vi "niRFUtil CONV Bit Stream to Number.vi"(3 "Length":i32 max=32, 4 "Index":i32, 5 "Bit Stream In":T1 min=0) -> (1 "Number":u32 max=16777215 format="%.0x", 2 "Bit Stream Out":T1 min=0)   [LabVIEW 2015, in "niRFUtil.lvlib"]
uses:
  niRFUtil.lvlib
  Includes/niRFUtil INC Bit Array.ctl
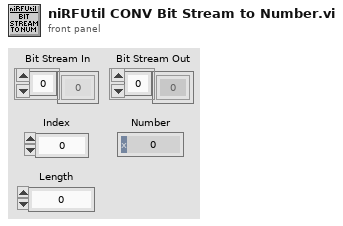
[diagram p1: front panel]
types:
  T1 = typedef "niRFUtil.lvlib/niRFUtil INC Bit Array.ctl" = i8[]
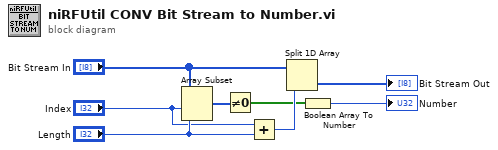
[diagram p0: block diagram]
diagram:
  n1 = Array Subset(array="Bit Stream In", index="Index", length="Length") -> (w3:T1)
  n2 = Not Equal To 0?(x=w3) -> (x != 0?=w2:bool[])
  n3 = Add(x="Index", y="Length") -> (x+y=w4:i32)
  n4 = Split 1D Array(array="Bit Stream In", index=w4) -> (second subarray=→"Bit Stream Out":T1)  [unwired: 1 out]
  n5 = Boolean Array To Number(Boolean array=w2) -> (number=→"Number":u32)
